vi "Create Testvi.vi"(8 "error in (no error)":errorcluster, 10 "Step Config":T1, 11 "Test Factory in":refnum<class "Test Factory.lvclass">) -> (0 "error out":errorcluster, 2 "Test Step.lvclass":refnum<class "Test Step.lvclass">, 3 "Test Factory out":refnum<class "Test Factory.lvclass">)   [LabVIEW 2021, in "Sequence Engine.lvlib" / "Test Factory.lvclass"]
uses:
  Test Factory.lvclass
  Test Step/Test Step.lvclass
  Test Config.ctl
  Test Cases/Measure/Measure.lvclass
  D:/Repositories/LabVIEW Codebase/Project Templates/Single Station PPL Template/Source/Modules/Sequence Engine/Classes/Test Step/Test Step.lvclass
  Test Factory.lvclass/Test Factory.ctl
  D:/Repositories/LabVIEW Codebase/Project Templates/Single Station PPL Template/Source/Modules/Sequence Engine/Classes/Test Cases/Measure/Measure.lvclass
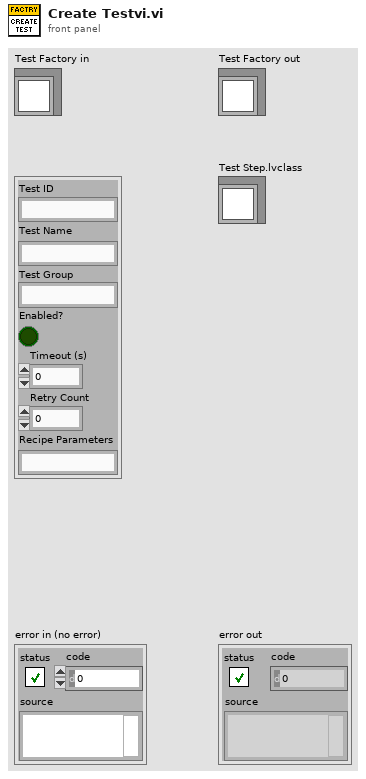
[diagram p1: front panel]
types:
  T1 = typedef "Sequence Engine.lvlib/Test Factory.lvclass/Test Config.ctl" = cluster{"Test ID":string, "Test Name":string, "Test Group":string, "Enabled?":bool, "Timeout (s)":u16, "Retry Count":u16, "Recipe Parameters":string}
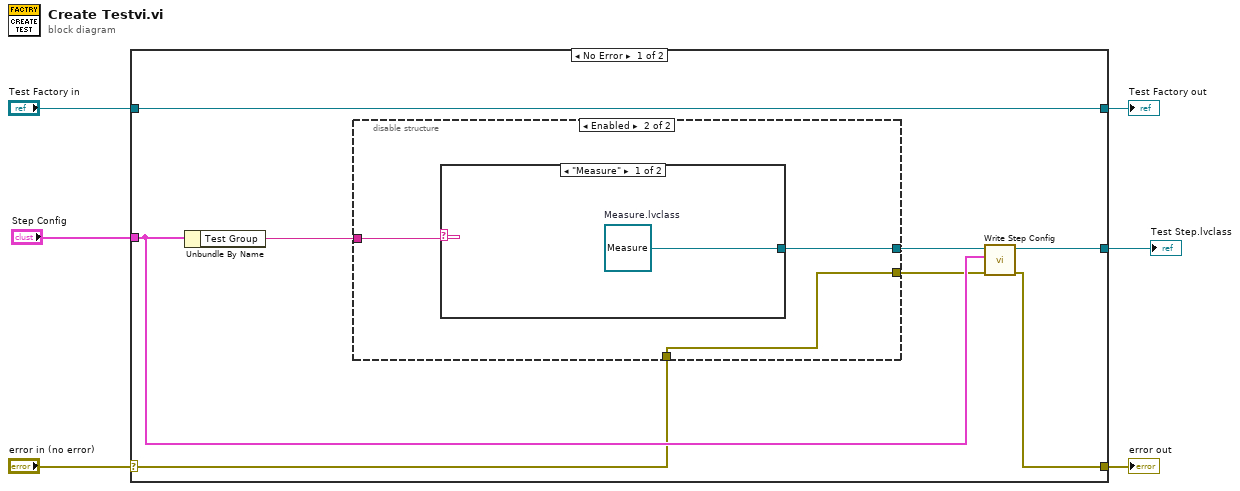
[diagram p0: block diagram]
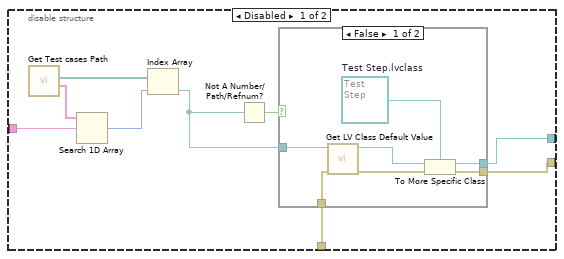
[diagram p2: hidden frame]
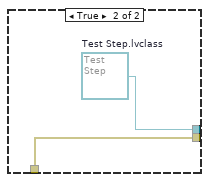
[diagram p3: hidden frame]
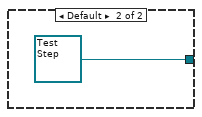
[diagram p4: hidden frame]
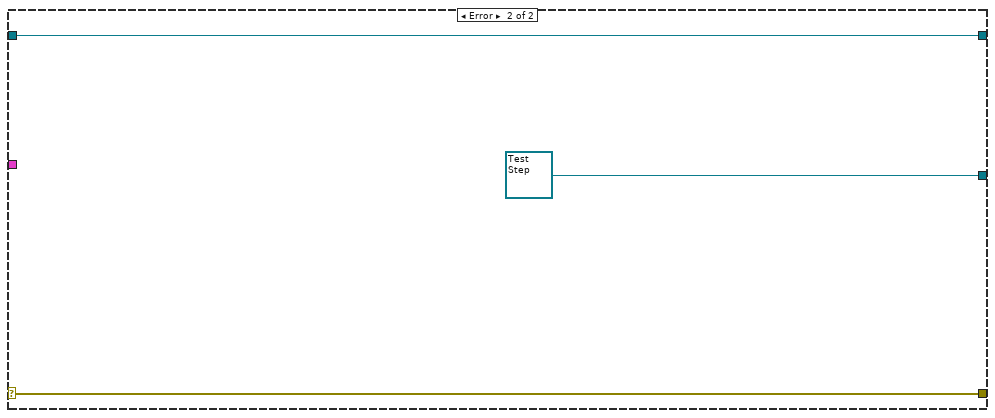
[diagram p5: hidden frame]
diagram:
  n1 = case shown="No Error" "error in (no error)" {
    selector: "error in (no error)" -> [w9 w40]
    tunnel: [w12 w40] -> w5
    tunnel: [w14 w39] -> w3
    tunnel: "Test Factory in" -> [w14 w39]
    tunnel: [w13 refnum<class "Test Step.lvclass"> refnum ("Test Step.lvclass")] -> w1
    tunnel: "Step Config" -> [w11 _]
    frame No Error {
      n2 = Unbundle By Name(w11) -> ("Test Group"=w10:string)
      n3 = disable-structure shown="Enabled" {
        disable-tunnel: w10 -> [w22 w33]
        disable-tunnel: w9 -> [w20 w34]
        disable-tunnel: [w19 w34] -> w8
        disable-tunnel: [w18 w35] -> w7
        frame Disabled {
          n4 = call "Get Test cases Path.vi"() -> ("folder names"=w23:string[], "Array"=w21:path[])  [unwired: 10 in]
          n5 = Search 1D Array(1D array=w23, element=w22) -> (index of element=w17:i32)  [unwired: 1 in]
          n6 = Index Array(array=w21, index=w17) -> (element=w15:path)
          n7 = Not A Number/Path/Refnum?(number/path/refnum=w15) -> (NaN/Path/Refnum?=w16:bool)
          n8 = case shown="False" w16 {
            tunnel: w20 -> [w30 w32]
            tunnel: w15 -> [w29 _]
            tunnel: [w26 w32] -> w19
            tunnel: [w25 w31] -> w18
            frame False {
              w24 = refnum<class "Test Step.lvclass"> refnum  # Test Step.lvclass
              n9 = call <vilib>:"Get LV Class Default Value.vi"("error in (no error)"=w30, "class path"=w29) -> ("error out"=w27:errorcluster, "object"=w28:refnum<class>)  [unwired: 8 in]
              n10 = To More Specific Class(target class=w24, reference=w28, error in=w27) -> (specific class reference=w25:refnum<class "Test Step.lvclass">, error out=w26:errorcluster)
            }
            frame True {
              w31 = refnum<class "Test Step.lvclass"> refnum  # Test Step.lvclass
            }
          }
        }
        frame Enabled {
          n11 = case shown="\"Measure\"" w33 {
            tunnel: [w36 refnum<class "Test Step.lvclass"> refnum ("Sequence Engine.lvlib:Test Step.lvclass")] -> w35
            frame "Measure" {
              w36 = refnum<class "Measure.lvclass"> refnum  # Measure.lvclass
            }
            frame Default {
            }
          }
        }
      }
      n12 = call-dynamic "Write Step Config.vi"("error in (no error)"=w8, "Step Config"=w11, "Test Step in"=w7) -> ("error out"=w12:errorcluster, "Test Step out"=w13:refnum<class "Test Step.lvclass">)  [unwired: 7 in]
    }
    frame Error {
    }
  }
  "error out" <- w5
  "Test Factory out" <- w3
  "Test Step.lvclass" <- w1
